vi "Modbus Master1.vi"() -> ()   [LabVIEW 2015]
uses:
  <vilib>/Modbus/subvis/Modbus API/Modbus API.lvclass/Modbus API.ctl
  <vilib>/Modbus/subvis/Transmission Data Unit (ADU)/Transmission Data Unit/Transmission Data Unit.lvclass/Transmission Data Unit.ctl
  <vilib>/Modbus/master/Data Access/Unit ID/Set Unit ID Property.vi
  <vilib>/Modbus/subvis/Transmission Data Unit (ADU)/Transmission Data Unit/Data Access/Unit ID/Write Unit ID.vi
  <vilib>/Modbus/subvis/Modbus API/Read Transmission Data Unit.vi
  <vilib>/Modbus/subvis/Modbus API/Write Transmission Data Unit.vi
  <vilib>/Modbus/master/Create Master Instance (Serial).vi
  <vilib>/Modbus/subvis/Transmission Data Unit (ADU)/Transmission Data Unit/Transmission Data Unit.lvclass
  <vilib>/Modbus/master/Modbus Master.lvclass
panel:
  out "Lamp 2":bool
  out "Read Register Slave 2":u16[](array[numeric])
  out "Lamp 1":bool
  out "LDR 2":u16
  out "LDR 1":u16
  out "LDR 2 (Volt)":dbl(knob) scale=0.0..5.0
  out "LDR 1 (Volt)":dbl(knob) scale=0.0..5.0
  out "Read Register Slave 1":u16[](array[numeric])
  in  "stop":bool
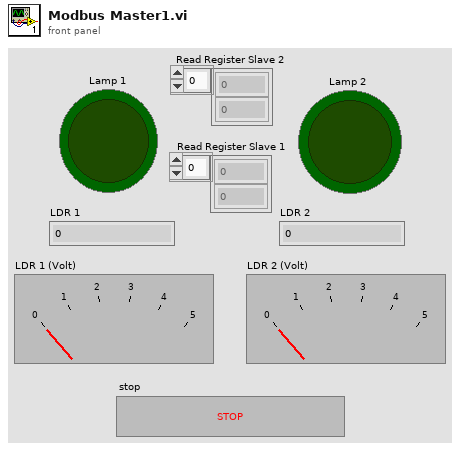
[diagram p1: front panel]
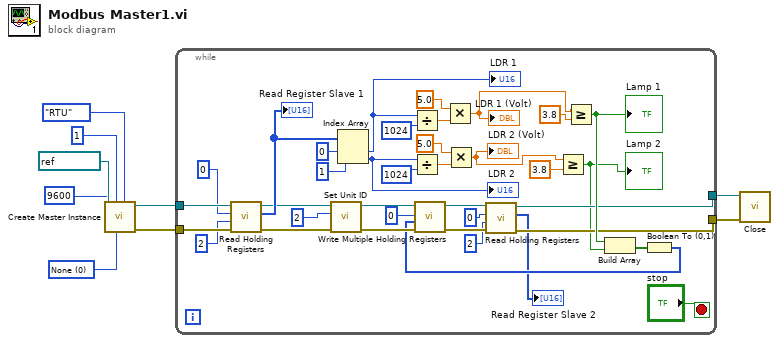
[diagram p0: block diagram]
diagram:
  w3 = u16 0 items=["None", "Odd", "Even"] ("parity (Even)")
  n1 = call-poly <vilib>:"Create Master Instance.vi"("serial type"=enum16{"RTU", "ASCII"}."RTU", "parity (Even)"=w3, "unit ID"=u8 1, "baud rate (9600)"=u32 9600, "VISA resource name"=refnum<visa-resource-name> "COM5") -> ("error out"=w8:errorcluster, "serial master instance"=w9:refnum<class "Modbus Master.lvclass">)  [unwired: 5 in]
  n2 = while {
    tunnel: w9 -> [w46]
    tunnel: w8 -> [w45]
    tunnel: [w15] -> w1
    tunnel: [w14] -> w2
    stop <- "stop" stop-if-true
    n3 = call-dynamic "Read Holding Registers.vi"("error in (no error)"=w45, "number of holding registers"=u16 2, "starting address"=u16 0, "Modbus master in"=w46) -> ("error out"=w29:errorcluster, "register values"=w41:u16[], "Modbus master out"=w30:refnum<class "Modbus Master.lvclass">)  [unwired: 5 in]
    "Read Register Slave 1" <- w41
    n4 = call <vilib>:"Set Unit ID.vi"("error in (no error)"=w29, "unit ID"=u8 2, "Modbus master in"=w30) -> ("error out"=w26:errorcluster, "Modbus master out"=w27:refnum<class "Modbus Master.lvclass">)  [unwired: 7 in]
    n5 = Index Array(array=w41, index #1=0 ("index"), index #2=1 ("index")) -> (element #1=w39:u16, element #2=w31:u16)
    "LDR 1" <- w39
    "LDR 2" <- w31
    n6 = Divide(x=w39, y=u16 1024) -> (x/y=w37:dbl)
    n7 = Divide(x=w31, y=u16 1024) -> (x/y=w34:dbl)
    n8 = Multiply(x=5.0, y=w37) -> (x*y=w24:dbl)
    "LDR 1 (Volt)" <- w24
    n9 = Multiply(x=5.0, y=w34) -> (x*y=w21:dbl)
    "LDR 2 (Volt)" <- w21
    n10 = Greater Or Equal?(x=w21, y=3.8) -> (x >= y?=w10:bool)
    "Lamp 2" <- w10
    n11 = Greater Or Equal?(x=w24, y=3.8) -> (x >= y?=w20:bool)
    "Lamp 1" <- w20
    n12 = Build Array(w20, w10) -> (w19:bool[])
    n13 = Boolean To (0,1)(Boolean=w19) -> (0, 1=w18:i16[])
    n14 = call-dynamic "Write Multiple Holding Registers.vi"("error in (no error)"=w26, "holding register values"=w18, "starting address"=u16 0, "Modbus master in"=w27) -> ("error out"=w16:errorcluster, "Modbus master out"=w17:refnum<class "Modbus Master.lvclass">)  [unwired: 6 in]
    n15 = call-dynamic "Read Holding Registers.vi"("error in (no error)"=w16, "number of holding registers"=u16 2, "starting address"=u16 0, "Modbus master in"=w17) -> ("error out"=w14:errorcluster, "register values"=→"Read Register Slave 2":u16[], "Modbus master out"=w15:refnum<class "Modbus Master.lvclass">)  [unwired: 5 in]
  }
  n16 = call-dynamic "Close.vi"("error in (no error)"=w2, "Modbus master in"=w1) -> ()  [unwired: 9 in, 1 out]
